vi "CSM - Request CSM to Post Message.vi"(6 "Without Reply?(F)":bool, 7 "Module Name":string, 8 "Error In (no error)":errorcluster, 9 "Target Module(\"\" by Default)":string, 10 "Arguments (\"\")":string, 11 "State":string="DoA") -> (0 "error out":errorcluster)   [LabVIEW 2014, in "Communicable State Machine.lvlib"]
doc: "Request JKISM to Post a message to JKISM specified. This is usually used in sub-loops with a JKISM for acting as a holistic module.\n\n<b>Inputs:</b>\n - <b>Status</b>: Message to post.\n - <b>Arguments (\"\")</b>: Argument of the message.\n - <b>Target Module</b>:Target CSM module name.\n - <b>Module Name</b>:Host Module Name\n - <b>Error In (no error)</b>: Error cluster\n\n<b>Outputs:</b>\n - <b>error out</b>: Error cluster"
uses:
  Communicable State Machine.lvlib
  _Support/JKISMQ/_CSMQFGVOPER.ctl
  _Support/Typedef/_Cross JKISM State Data.ctl
  _Support/Typedef/_CSM_MSG_TYPE.ctl
  _Support/Typedef/_Cross JKISM State Response.ctl
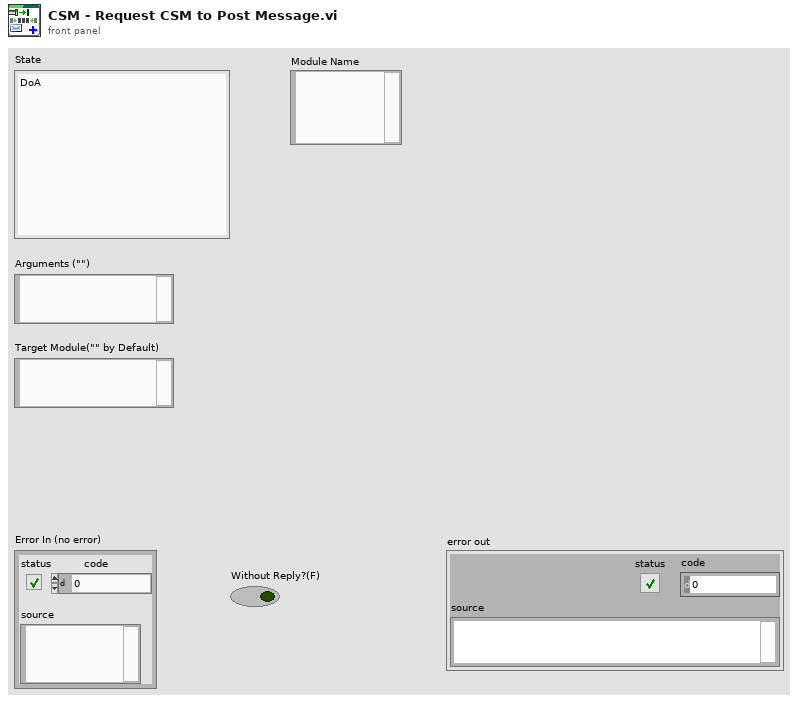
[diagram p1: front panel]
types:
  T1 = typedef "Communicable State Machine.lvlib/_CSM_MSG_TYPE.ctl" = enum16{"Sync Message(-@)", "Async Message(->)", "Async without Response(->|)", "Async Response", "Broadcast(-><status>)", "Broadcast(-><interrupt>)", "Request to Post Message", "Request to Post Message without Reply", "Request to Publish Status"}
  T2 = typedef "Communicable State Machine.lvlib/_Cross JKISM State Data.ctl" = cluster{"Msg Type":T1, "state":string, "args":string, "source":string, "RespQ":refnum<queue>, "Pre-State":string, "Arg-State":string, "Target":string}
  T3 = typedef "Communicable State Machine.lvlib/_CSMQFGVOPER.ctl" = enum16{"Get By Name", "List", "Check If Name Exists", "Release", "Module Status", "Create Status Event Handler", "Destroy Status Event Handler"}
  T4 = typedef "Communicable State Machine.lvlib/_CSMQ.ctl" = cluster{"Module Name":string, "Queue":refnum<queue>, "Locked Status":refnum<data-value>, "Mode":T5, "User Event":refnum<user-event>, "Queue Count":i32, "Status Change Event":refnum<user-event>}
  T5 = typedef "Communicable State Machine.lvlib/_CSM_MODE.ctl" = enum16{"Stand Alone", "CSM", "Action Worker"}
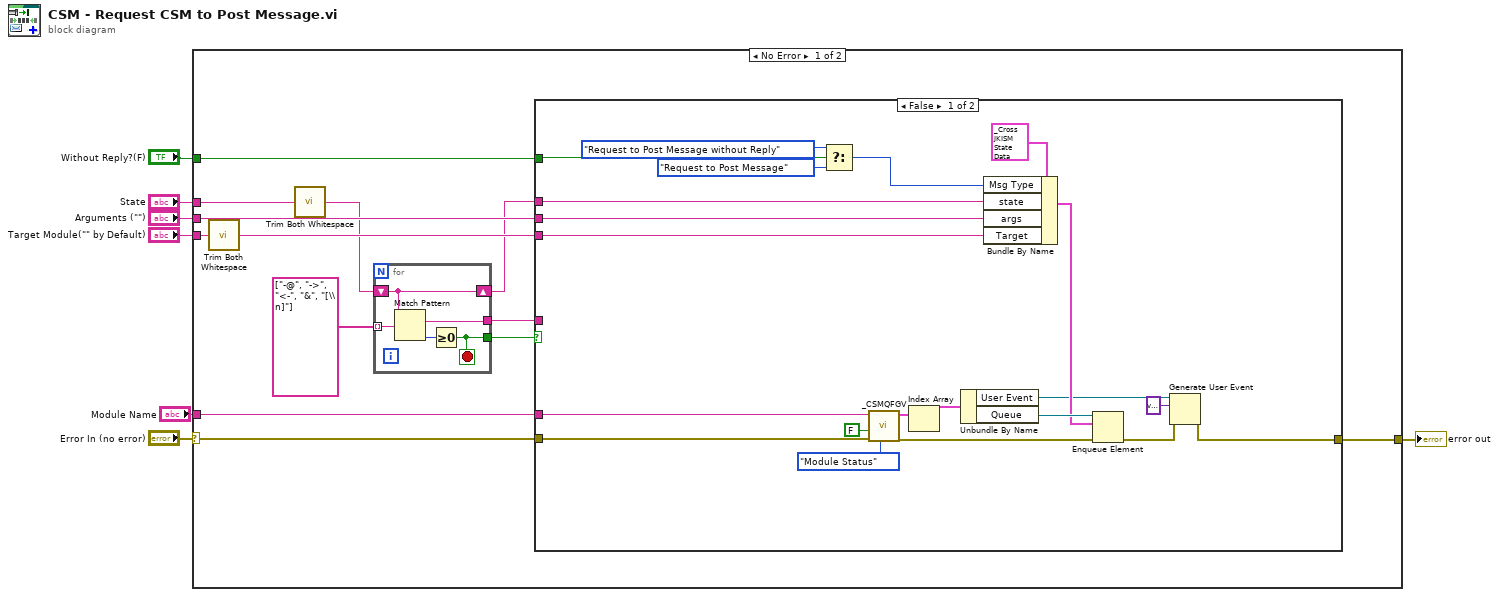
[diagram p0: block diagram]
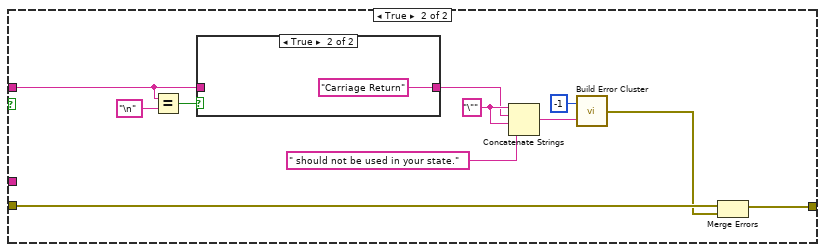
[diagram p2: hidden frame]
diagram:
  n1 = case shown="No Error" "Error In (no error)" {
    selector: "Error In (no error)" -> [w18 w60]
    tunnel: "State" -> [w15 _]
    tunnel: [w19 w60] -> w5
    tunnel: "Arguments (\"\")" -> [w16 _]
    tunnel: "Target Module(\"\" by Default)" -> [w20 _]
    tunnel: "Module Name" -> [w14 _]
    tunnel: "Without Reply?(F)" -> [w13 _]
    frame No Error {
      n2 = call "Trim Both Whitespace.vi"("string"=w20) -> ("trimmed string"=w17:string)  [unwired: 1 in]
      n3 = call "Trim Both Whitespace.vi"("string"=w15) -> ("trimmed string"=w8:string)  [unwired: 1 in]
      n4 = for {
        shift-right: [w59] -> w11
        shift-left: w8 -> [w59]
        tunnel: string[] ["-@", "->", "<-", "&", "[\\n]"] -> [w58] mode=indexing
        tunnel: [w56] -> w9
        tunnel: [w55] -> w10
        stop <- w55 stop-if-true
        n5 = Match Pattern(string=w59, regular expression=w58) -> (match substring=w56:string, offset past match=w57:i32)  [unwired: 1 in, 2 out]
        n6 = Greater Or Equal To 0?(x=w57) -> (x >= 0?=w55:bool)
      }
      n7 = case shown="False" w10 {
        tunnel: w16 -> [w34 _]
        tunnel: w17 -> [w33 _]
        tunnel: [w23 w44] -> w19
        tunnel: w18 -> [w31 w45]
        tunnel: w11 -> [w35 _]
        tunnel: w9 -> [_ w42]
        tunnel: w14 -> [w29 _]
        tunnel: w13 -> [w27 _]
        frame False {
          n8 = Select(t=_CSM_MSG_TYPE."Request to Post Message without Reply" ("Msg Type"), s=w27, f=_CSM_MSG_TYPE."Request to Post Message" ("Msg Type")) -> (s? t:f=w24:T1)
          n9 = call "_CSMQFGV.vi"("Operation"=_CSMQFGVOPER."Module Status", "Error in"=w31, "create if not found? (T)"=FALSE, "Name(\"\" to use uuid) in"=w29) -> ("Error out"=w32:errorcluster, "Array"=w40:T4[])  [unwired: 4 in, 2 out]
          n10 = Index Array(array=w40) -> (element=w39:T4)  [unwired: 1 in]
          n11 = Unbundle By Name(w39) -> ("User Event"=w22:refnum<user-event>, "Queue"=w38:refnum<queue>)
          n12 = Bundle By Name(cluster=T2 {"Msg Type"=enum."Sync Message(-@)", "state"="", "args"="", "source"="", "RespQ"=refnum, "Pre-State"="", "Arg-State"="", "Target"=""} ("element"), "Msg Type"=w24, "state"=w35, "args"=w34, "Target"=w33) -> (w36:T2)
          n13 = Enqueue Element(queue=w38, element=w36, error in (no error)=w32) -> (error out=w30:errorcluster)  [unwired: 1 in, 2 out]
          n14 = Generate User Event(user event=w22, event data cluster=variant ("event data"), error in=w30) -> (error out=w23:errorcluster)  [unwired: 1 in, 1 out]
        }
        frame True {
          w49 = "\"" ("string")
          n15 = Equal?(x=w42, y="\n" ("regular expression")) -> (x = y?=w46:bool)
          n16 = case shown="True" w46 {
            tunnel: [w53 "Carriage Return" ("State")] -> w48
            tunnel: w42 -> [w53 _]
            frame False {
            }
            frame True {
            }
          }
          n17 = Concatenate Strings(w49, w48, w49, " should not be used in your state." ("String to Prepend to source (\"\")")) -> (w50:string)
          n18 = call "Build Error Cluster.vi"("String to Prepend to source (\"\")"=w50, "code"=-1) -> ("error out"=w43:errorcluster)
          n19 = Merge Errors(w45, w43) -> (w44:errorcluster)
        }
      }
    }
    frame Error {
    }
  }
  "error out" <- w5
